vi "111.vi"(0 "停止?":bool, 2 "Baudrate":u32(ring)=1000 caption="K" items=["10"=10, "20"=20, "50"=50, "100"=100, "125"=125, "250"=250, "500"=500, "800"=800, "1000"=1000], 3 "CANPort":string(combo)="CAN1") -> (8 "成功？":bool)   [LabVIEW 2010]
uses:
  全局量/全局_配置.vi
panel:
  out "数组":u8[](array[numeric]) format="%x"
  out "字节数":i32
  out "Error out":errorcluster {"code" format="%.0x"}
  in  "ReadTimeOut":u32=3000 caption="ms"
  in  "Synchronization":i32(ring)=1 items=["Synchronization"=1, "Asynchronization"=0]
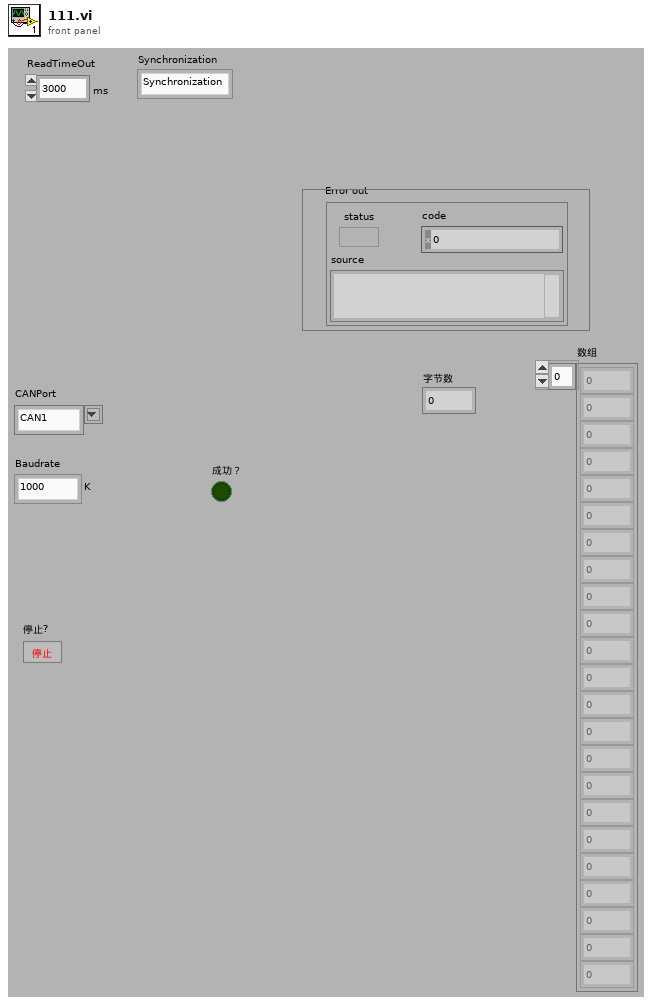
[diagram p1: front panel]
types:
  T1 = cluster{"Internal":u32, "InternalHigh":u32, "Offset":u32, "OffsetHigh":u32, "hEvent":u32}
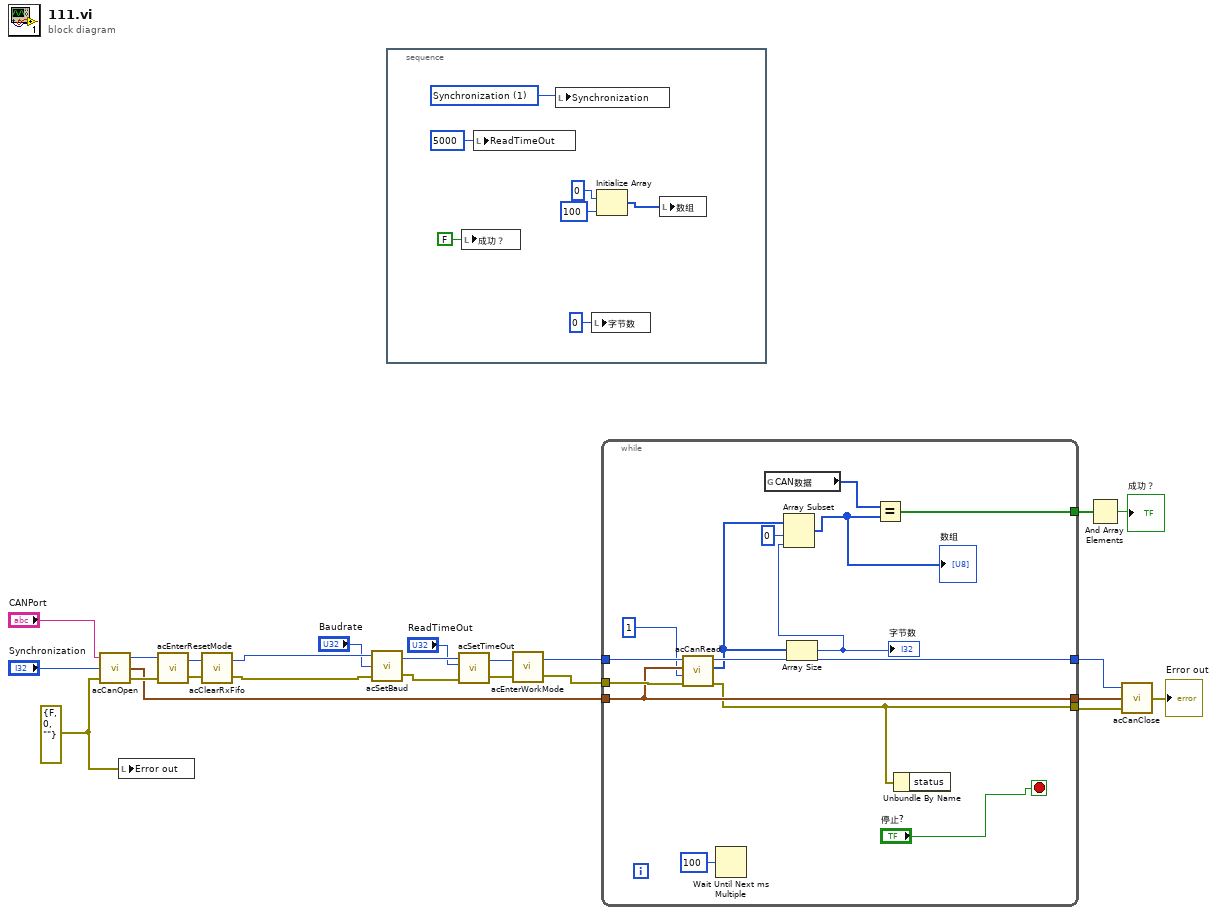
[diagram p0: block diagram]
diagram:
  w17 = errorcluster {"status"=FALSE, "code"=0, "source"=""} ("Error in")
  n1 = call "acCanOpen.vi"("Error in"=w17, "Synchronization"="Synchronization", "CANPort"="CANPort") -> ("Error out"=w19:errorcluster, "Overlapped"=w4:T1, "Handle"=w20:u32)
  n2 = local write "Error out"(w17) -> ()
  n3 = call "acEnterResetMode.vi"("Error in"=w19, "Handle  in"=w20) -> ("Error out"=w12:errorcluster, "Handle out"=w11:u32)
  n4 = call "acClearRxFifo.vi"("Error in"=w12, "Handle  in"=w11) -> ("Error out"=w9:errorcluster, "Handle out"=w10:u32)
  n5 = call "acSetBaud.vi"("Error in"=w9, "Baudrate"="Baudrate", "Handle  in"=w10) -> ("Error out"=w14:errorcluster, "Handle out"=w15:u32)
  n6 = stacked-sequence {
    frame #0 {
      w29 = 1 items=["Synchronization"=1, "Asynchronization"=0] ("Synchronization")
      n7 = local write "成功？"(FALSE ("成功？")) -> ()
      n8 = local write "ReadTimeOut"(u32 5000 ("ReadTimeOut")) -> ()
      n9 = local write "Synchronization"(w29) -> ()
      n10 = local write "字节数"(0 ("字节数")) -> ()
      n11 = Initialize Array(u8 0 ("字节数"), 100 ("维数大小")) -> (w25:u8[])
      n12 = local write "数组"(w25) -> ()
    }
  }
  n13 = call "acSetTimeOut.vi"("Error in"=w14, "Read TimeOut"="ReadTimeOut", "Handle  in"=w15) -> ("Error out"=w7:errorcluster, "Handle out"=w8:u32)  [unwired: 1 in]
  n14 = call "acEnterWorkMode.vi"("Error in"=w7, "Handle  in"=w8) -> ("Error out"=w5:errorcluster, "Handle out"=w6:u32)
  n15 = while {
    tunnel: w6 -> [w44]
    tunnel: w5 -> [w45]
    tunnel: [w42] -> w21
    tunnel: [w40] -> w23
    tunnel: w4 -> [w43]
    tunnel: [w43] -> w22
    tunnel: [w36] -> w2
    stop <- "停止?" stop-if-true
    n16 = call "acCanRead.vi"("Error in"=w45, "ReadCount"=u32 1 ("接收CAN帧数 2"), "Overlapped"=w43, "Handle  in"=w44) -> ("Error out"=w42:errorcluster, "MSG"=w34:u8[], "Handle out"=w40:u32)  [unwired: 1 out]
    n17 = Wait Until Next ms Multiple(millisecond multiple=u32 100) -> ()  [unwired: 1 out]
    n18 = global read "全局_配置.vi" "CAN数据"() -> (w38:u8[])
    n19 = Array Size(array=w34) -> (size(s)=w32:i32)
    "字节数" <- w32
    n20 = Array Subset(array=w34, index=0 ("索引"), length=w32) -> (w33:u8[])
    "数组" <- w33
    n21 = Equal?(x=w38, y=w33) -> (x = y?=w36:bool[])
    n22 = Unbundle By Name(w42) -> ()  [unwired: 1 out]
  }
  n23 = And Array Elements(Boolean array=w2) -> (logical AND=→"成功？":bool)
  n24 = call "acCanClose.vi"("Error in"=w21, "Overlapped"=w22, "Handle  in"=w23) -> ("Error out"=→"Error out":errorcluster)
